vi "State Exit.vi"(8 "error in (no error)":errorcluster, 11 "View Model":T1) -> (0 "error out":errorcluster, 3 "View Model":T1)   [LabVIEW 2017]
doc: "Process finish an actuall elevator controller state."
uses:
  View Model/Controls/View Model.ctl
  View Model/Controls/Shared Model.ctl
  Error Handler/Controls/Error Model.ctl
  Error Handler/Controls/Error Data.ctl
  Error Handler/Controls/Error Level.ctl
  Configuration/Controls/Config Model.ctl
  Configuration/Controls/Config Data Record.ctl
  Configuration/Controls/Config Command.ctl
  Controls/Control Model.ctl
  Controls/Elevator Location.ctl
  Controls/Elevator Status.ctl
  Controls/Control Event.ctl
  Controls/Control CMD.ctl
  Controls/Controller - Overhead.ctl
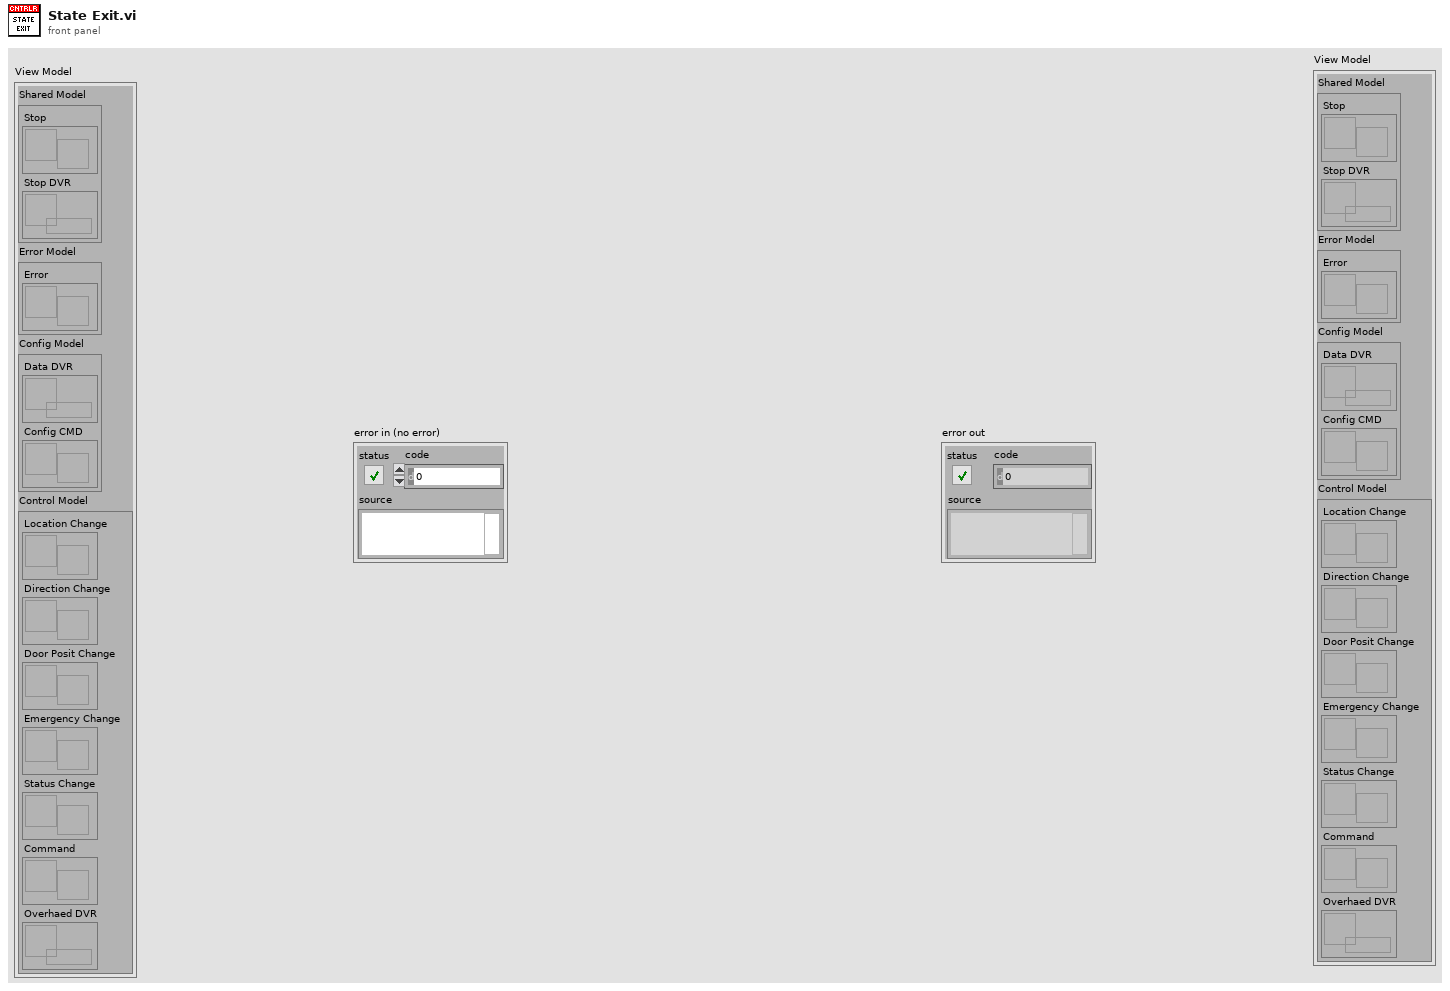
[diagram p1: front panel]
types:
  T1 = typedef "View Model.ctl" = cluster{"Shared Model":T2, "Error Model":T3, "Config Model":T4, "Control Model":T5}
  T2 = typedef "Shared Model.ctl" = cluster{"Stop":refnum<user-event>, "Stop DVR":refnum<data-value>}
  T3 = typedef "Error Model.ctl" = cluster{"Error":refnum<user-event>}
  T4 = typedef "Config Model.ctl" = cluster{"Data DVR":refnum<data-value>, "Config CMD":refnum<user-event>}
  T5 = typedef "Control Model.ctl" = cluster{"Location Change":refnum<user-event>, "Direction Change":refnum<user-event>, "Door Posit Change":refnum<user-event>, "Emergency Change":refnum<user-event>, "Status Change":refnum<user-event>, "Command":refnum<user-event>, "Overhaed DVR":refnum<data-value>}
  T6 = typedef "Elevator Status.ctl" = enum16{"No Request", "Initial", "Wait for 1st Request", "Start and Move", "Continue Move", "Analysis", "Stop at Floor", "Open/Close Door", "Emergency Call", "Terminate"}
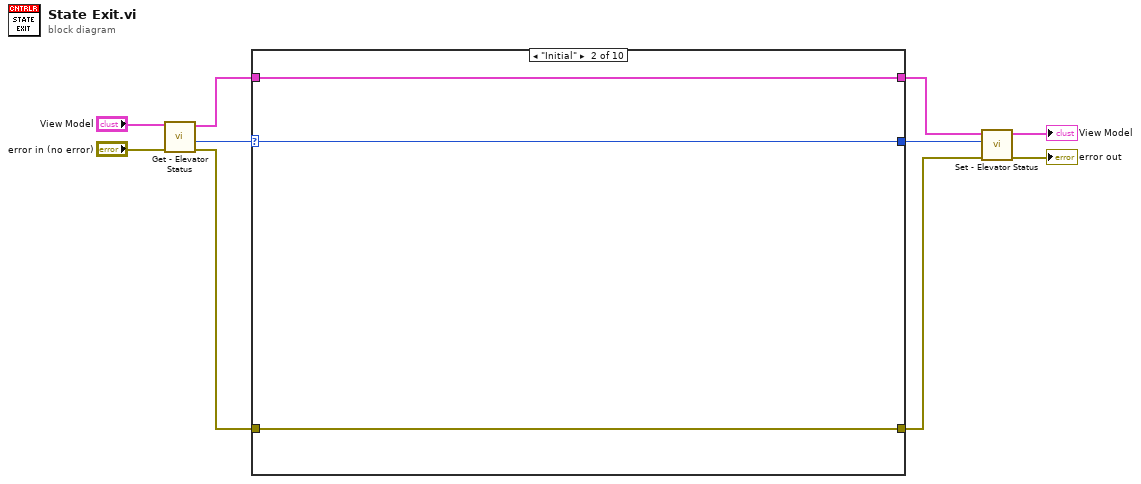
[diagram p0: block diagram]
diagram:
  n1 = call "Get - Elevator Status.vi"("error in (no error)"="error in (no error)", "View Model"="View Model") -> ("error out"=w2:errorcluster, "Next Status"=w9:T6, "View Model"=w8:T1)  [unwired: 6 in, 1 out]
  n2 = case shown="\"Initial\"" w9 {
    selector: w9 -> [_ w13 _ _ _ _ _ _ _ _]
    tunnel: w8 -> [w12 w15 w17 w19 w21 w23 w25 w27 w29 w31]
    tunnel: [w12 w15 w17 w19 w21 w23 w25 w27 w29 w31] -> w7
    tunnel: w2 -> [w11 w14 w16 w18 w20 w22 w24 w26 w28 w30]
    tunnel: [w11 w14 w16 w18 w20 w22 w24 w26 w28 w30] -> w3
    tunnel: [_ w13 _ _ _ _ _ _ _ _] -> w1
    frame "No Request", Default {
    }
    frame "Initial" {
    }
    frame "Wait for 1st Request" {
    }
    frame "Start and Move" {
    }
    frame "Continue Move" {
    }
    frame "Analysis" {
    }
    frame "Stop at Floor" {
    }
    frame "Open/Close Door" {
    }
    frame "Emergency Call" {
    }
    frame "Terminate" {
    }
  }
  n3 = call "Set - Elevator Status.vi"("error in (no error)"=w3, "Current Status"=w1, "View Model"=w7) -> ("error out"=→"error out":errorcluster, "View Model"=→"View Model":T1)  [unwired: 7 in]
